vi "QR2POS.vi"(10 "QR_string":string) -> (0 "Start Out Point":dbl[](array[numeric])=[0.0, 0.1725], 1 "Start Front":dbl[](array[numeric])=[0.0, 0.3925, 0.0], 2 "Start POS":dbl[](array[numeric]), 3 "heading":dbl, 4 "Block Array":dbl[][](array[numeric]), 5 "X/Y/Z":dbl[](array[numeric]))   [LabVIEW 2018]
uses:
  b469bd63-f4ec-42e9-9963-4ddcccfafac0.vi
  <vilib>/Analysis/coordinate.llb/2D Cartesian Coordinate Rotation (Scalar).vi
  <vilib>/Array/Sort 2D Array - Pop Stack.vi
  <vilib>/Array/Sort 2D Array - Push Stack.vi
  b469bd63-f4ec-42e9-9963-4ddcccfafac0.vi/234f02b5-400b-4322-a671-b314699ba740.vi
  b469bd63-f4ec-42e9-9963-4ddcccfafac0.vi/9389aebd-445b-454c-9412-fcfb9eb6e520.vi
  <vilib>/Analysis/NI_AALPro.lvlib
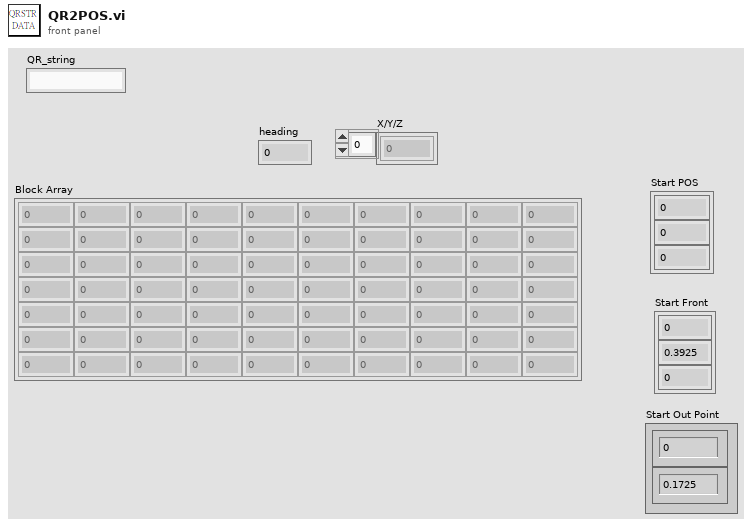
[diagram p1: front panel]
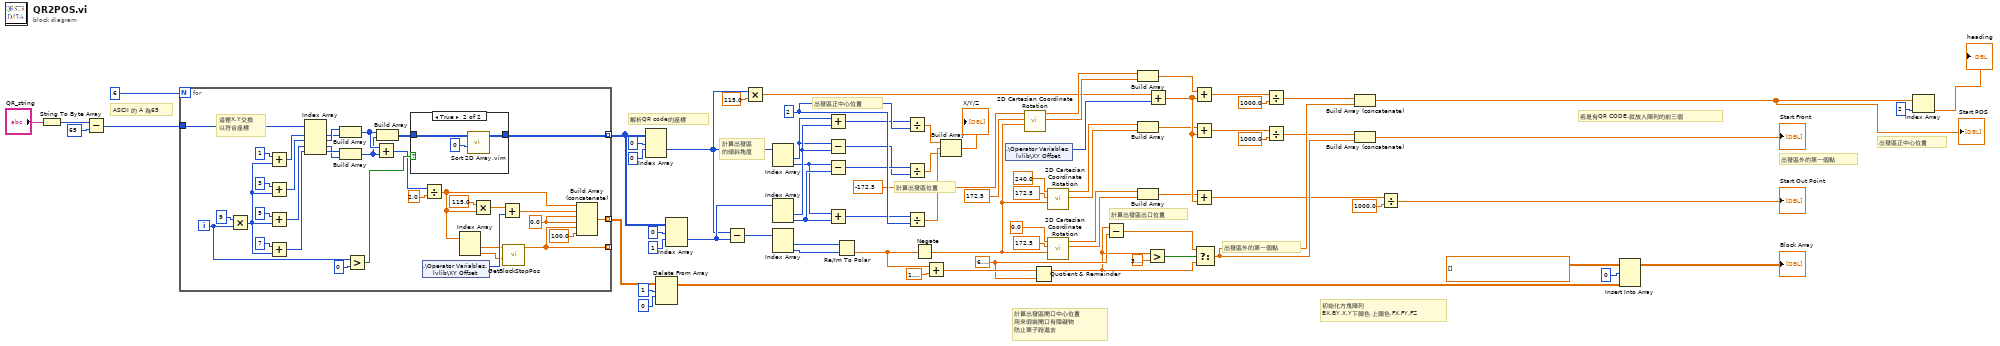
[diagram p0: block diagram]
diagram:
  w72 = 2 ("y")
  w14 = 6.283185307179586
  # "若是有QR CODE,就放入陣列的前三個"
  # "計算出發區開口中心位置\n用來假裝開口有障礙物\n防止車子跑進去"
  # "出發區外的第一個點"
  # "出發區正中心位置"
  # "初始化方塊陣列\nBX,BY,X,Y下顏色,上顏色,FX,FY,FZ"
  # "出發區外的第一個點"
  # "出發區正中心位置"
  # "計算出發區出口位置"
  # "計算出發區位置"
  # "計算出發區\n的傾斜角度"
  # "解析QR code的座標"
  # "ASCII 的 A 為65"
  n1 = String To Byte Array(string="QR_string") -> (unsigned byte array=w33:u8[])
  n2 = Subtract(x=w33, y=65) -> (x-y=w31:i32[])
  n3 = for {
    N: 6 -> [_]
    tunnel: w31 -> [w112]
    tunnel: [w101] -> w27 mode=indexing
    tunnel: [w80] -> _ mode=indexing
    tunnel: [w78] -> w56 mode=indexing
    i -> [w99]
    w84 = 0.0
    # "這裡X,Y交換\n以符合座標"
    n4 = Multiply(x=9, y=w99) -> (x*y=w106:i32)
    n5 = Add(x=1 ("index"), y=w106) -> (x+y=w105:i32)
    n6 = Add(x=3 ("index"), y=w106) -> (x+y=w104:i32)
    n7 = Add(x=5 ("index"), y=w106) -> (x+y=w103:i32)
    n8 = Add(x=7 ("index"), y=w106) -> (x+y=w102:i32)
    n9 = Index Array(array=w112, index #1=w105, index #2=w104, index #3=w103, index #4=w102) -> (element #1=w95:i32, element #2=w96:i32, element #3=w93:i32, element #4=w94:i32)
    n10 = Build Array(w96, w95) -> (w92:i32[])
    n11 = Build Array(w94, w93) -> (w89:i32[])
    n12 = Greater?(x=w99, y=0) -> (0:w100:bool)
    n13 = Add(x=w92, y=w89) -> (x+y=w91:i32[])
    n14 = Build Array(w92, w89) -> (w97:i32[][])
    n15 = case shown="True" w100 {
      tunnel: w97 -> [w113 w116]
      tunnel: [w113 w114] -> w101
      frame False {
      }
      frame True {
        n16 = call "Sort 2D Array.vim"("index"=0, "2D array"=w116) -> ("sorted 2D array"=w114:i32[][])  [unwired: 8 in, 1 out]
      }
    }
    n17 = shared-variable ".\\Operator Variables.lvlib\\XY Offset"() -> (w85:i16)  [unwired: 1 in, 1 out]
    n18 = Divide(x=w91, y=2.0) -> (x/y=w79:dbl[])
    n19 = Index Array(array=w79) -> (element #1=w82:dbl, element #2=w81:dbl)  [unwired: 2 in]
    n20 = Multiply(x=115.0, y=w79) -> (x*y=w86:dbl[])
    n21 = Add(x=w86, y=w85) -> (x+y=w87:dbl[])
    n22 = call "GetBlockStopPos.vi"("YB"=w81, "XB"=w82) -> ("Array"=w80:dbl[])  [unwired: 8 in, 1 out]
    n23 = Build Array (concatenate)(w79, w87, w84, w84, w80, 100.0) -> (w78:dbl[])
  }
  n24 = Index Array(array=w27, index (dim 0)=0 ("index (page)"), index (dim 1)=0 ("disabled index (row)")) -> (element=w61:i32[])  [unwired: 1 in]
  n25 = Delete From Array(array=w56, length=1, index (row)=0) -> (array with subset deleted=w51:dbl[][])  [unwired: 1 in, 1 out]
  n26 = Index Array(array=w27, index (dim 0)=0 ("index (page)"), index (dim 1)=1 ("disabled index (row)")) -> (element=w62:i32[])  [unwired: 1 in]
  n27 = Subtract(x=w61, y=w62) -> (x-y=w24:i32[])
  n28 = Multiply(x=w61, y=115.0) -> (x*y=w9:dbl[])
  n29 = Index Array(array=w61) -> (element #1=w66:i32, element #2=w67:i32)  [unwired: 2 in]
  n30 = Index Array(array=w62) -> (element #1=w68:i32, element #2=w69:i32)  [unwired: 2 in]
  n31 = Index Array(array=w24) -> (element #1=w23:i32, element #2=w22:i32)  [unwired: 2 in]
  n32 = Add(x=w66, y=w68) -> (x+y=w70:i32)
  n33 = Subtract(x=w66, y=w68) -> (x-y=w63:i32)
  n34 = Subtract(x=w67, y=w69) -> (x-y=w64:i32)
  n35 = Add(x=w67, y=w69) -> (x+y=w71:i32)
  n36 = Re/Im To Polar(2:w22, 3:w23) -> (0:w2:dbl)  [unwired: 1 out]
  n37 = Divide(x=w70, y=w72) -> (x/y=w73:dbl)
  n38 = Divide(x=w64, y=w63) -> (x/y=w74:dbl)
  n39 = Divide(x=w71, y=w72) -> (x/y=w75:dbl)
  n40 = Negate(x=w2) -> (-x=w43:dbl)
  n41 = Add(x=w2, y=1.5707963267948966) -> (x+y=w18:dbl)
  n42 = Build Array(w73, w75, w74) -> (→"X/Y/Z":dbl[])
  n43 = shared-variable ".\\Operator Variables.lvlib\\XY Offset"() -> (w8:i16)  [unwired: 1 in, 1 out]
  n44 = call-poly <vilib>:"2D Cartesian Coordinate Rotation.vi"("theta"=w43, "y"=172.5, "x"=-172.5) -> ("y out"=w11:dbl, "x out"=w12:dbl)  [unwired: 6 in, 1 out]
  n45 = Quotient & Remainder(x=w18, y=w14) -> (x-y*floor(x/y)=w13:dbl)  [unwired: 1 out]
  n46 = call-poly <vilib>:"2D Cartesian Coordinate Rotation.vi"("theta"=w43, "y"=172.5, "x"=240.0) -> ("y out"=w4:dbl, "x out"=w5:dbl)  [unwired: 6 in, 1 out]
  n47 = call-poly <vilib>:"2D Cartesian Coordinate Rotation.vi"("theta"=w43, "y"=172.5, "x"=0.0) -> ("y out"=w41:dbl, "x out"=w40:dbl)  [unwired: 6 in, 1 out]
  n48 = Subtract(x=w13, y=w14) -> (x-y=w15:dbl)
  n49 = Build Array(w12, w11) -> (w10:dbl[])
  n50 = Build Array(w5, w4) -> (w3:dbl[])
  n51 = Build Array(w40, w41) -> (w44:dbl[])
  n52 = Greater?(x=w13, y=3.141592653589793) -> (0:w16:bool)
  n53 = Add(x=w9, y=w8) -> (x+y=w45:dbl[])
  n54 = Add(x=w10, y=w45) -> (x+y=w37:dbl[])
  n55 = Add(x=w3, y=w45) -> (x+y=w35:dbl[])
  n56 = Add(x=w44, y=w45) -> (x+y=w46:dbl[])
  n57 = Select(t=w15, s=w16, f=w13) -> (s? t:f=w48:dbl)
  n58 = Divide(x=w37, y=1000.0) -> (x/y=w65:dbl[])
  n59 = Divide(x=w35, y=1000.0) -> (x/y=w36:dbl[])
  n60 = Build Array (concatenate)(w65, w48) -> (w58:dbl[])
  "Start POS" <- w58
  n61 = Build Array (concatenate)(w36, w48) -> (→"Start Front":dbl[])
  n62 = Divide(x=w46, y=1000.0) -> (x/y=→"Start Out Point":dbl[])
  n63 = Insert Into Array(array=dbl[][] [], index (row)=0, new element=w51) -> (→"Block Array":dbl[][])  [unwired: 1 in]
  n64 = Index Array(array=w58, index=2) -> (element=→"heading":dbl)
